vi "Disable_and_Start.vi"(0 "System data in":T1, 5 "Data":variant, 7 "Wash Options In":refnum<vi>, 9 "Wash Entry":refnum<vi>, 11 "error in (no error)":errorcluster) -> (4 "System data out":T1, 15 "error out":errorcluster)   [LabVIEW 2023]
doc: "This VI ddiables the car wash options and starts the washing process"
uses:
  Controls/System_Data.ctl
  Controls/Wash Options.ctl
  Controls/State.ctl
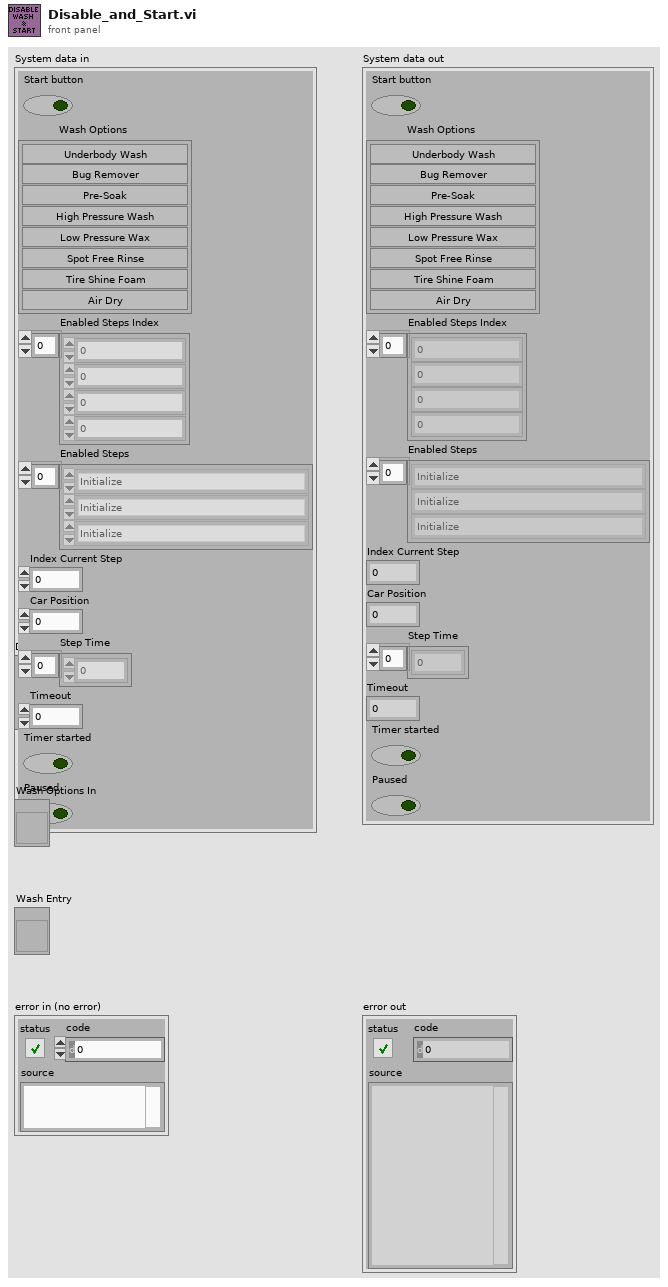
[diagram p1: front panel]
types:
  T1 = typedef "System_Data.ctl" = cluster{"Start button":bool, "Wash Options":T2, "Enabled Steps Index":i32[], "Enabled Steps ":T3[], "Index Current Step":i32, "Car Position":u8, "Step Time":dbl[], "Timeout":i32, "Timer started":bool, "Paused":bool}
  T2 = typedef "Wash Options.ctl" = cluster{"Underbody Wash":bool, "Bug Remover":bool, "Pre-Soak":bool, "High Pressure Wash":bool, "Low Pressure Wax":bool, "Spot Free Rinse":bool, "Tire Shine Foam":bool, "Air Dry":bool}
  T3 = typedef "State.ctl" = enum16{"Initialize", "Wait for Something", "Step Completed", "Save Wash Options", "Start Process", "Car Position", "Order Steps to follow", "Underbody Wash", "Bug Remover", "Pre-Soak", "High Pressure Wash", "Low Pressure Wax", "Spot Free Rinse", "Tire Shine Foam", "Air Dry", "Vehicle out of position", "Exit", "Process Complete", "Stop Application"}
  T4 = enum8{"Enabled", "Disabled", "Disabled and Grayed Out"}
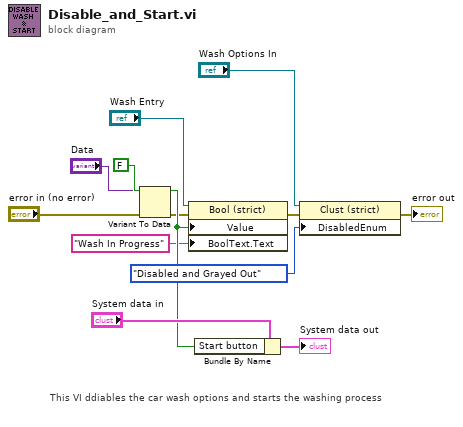
[diagram p0: block diagram]
diagram:
  # "This VI ddiables the car wash options and starts the washing process"
  n1 = Variant To Data(error in="error in (no error)", type=FALSE, Variant="Data") -> (data=w7:bool, error out=w5:errorcluster)
  n2 = property class="Bool (strict)"(reference="Wash Entry", error in=w5, "Value"=w7, "BoolText.Text"="Wash In Progress" ("Boolean Text.Text")) -> (error out=w3:errorcluster)  [unwired: 1 out]
  n3 = Bundle By Name(cluster="System data in", "Start button"=w7) -> (→"System data out":T1)
  n4 = property class="Clust (strict)"(reference="Wash Options In", error in=w3, "DisabledEnum"=T4."Disabled and Grayed Out" ("Disabled")) -> (error out=→"error out":errorcluster)  [unwired: 1 out]
